vi "SelectMouseRoi.vi"(6 "Refnum in":T1, 7 "Select mouse":bool, 10 "File Path for Mouse Mask":path=path "C:/PassiveRotationTask/MousePositionMask.bmp", 11 "MouseRoi":T1) -> (3 "MouseRoi Out":T1)   [LabVIEW 2013]
uses:
  <vilib>/vision/Image Controls.llb/IMAQ Image.ctl
  <vilib>/vision/NI_Vision_Development_Module.lvlib
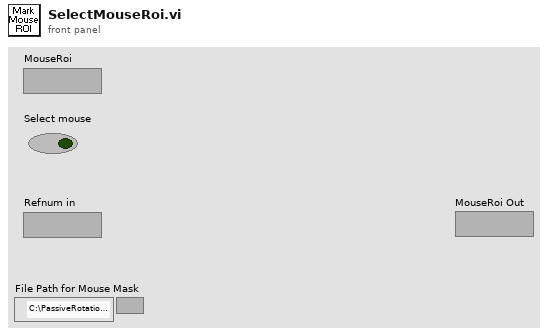
[diagram p1: front panel]
types:
  T1 = typedef "IMAQ Image.ctl" = refnum<image>
  T2 = typedef "ROI Descriptor" = cluster{"Global Rectangle":i32[], "Contours":cluster{"ID":enum32{"External", "Internal"}, "Type":u32, "Coordinates":i32[]}[]}
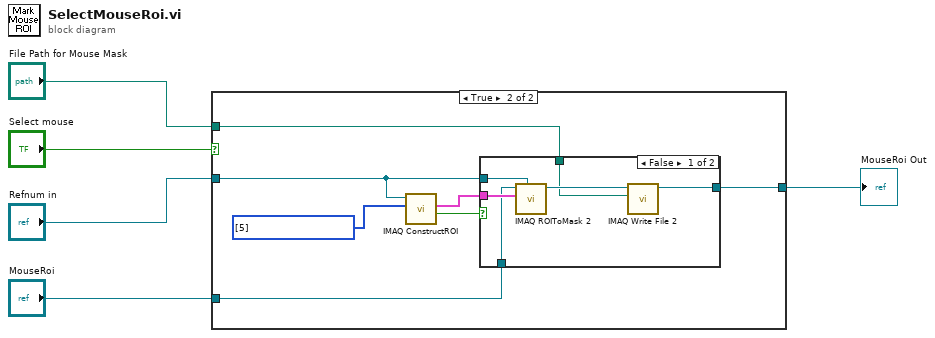
[diagram p0: block diagram]
diagram:
  n1 = case shown="True" "Select mouse" {
    tunnel: "Refnum in" -> [_ w11]
    tunnel: "File Path for Mouse Mask" -> [_ w9]
    tunnel: "MouseRoi" -> [w6 w8]
    tunnel: [w6 w7] -> w1
    frame False {
    }
    frame True {
      w13 = u32[] [5] items=["No Selection", "Point", "Line", "Rectangle", "Oval", "Polygon", "Freehand Region", "Annulus", "Zoom", "Pan", "Broken Line", "Freehand Line", "Rotated Rectangle"] ("Tools")
      n2 = call "IMAQ ConstructROI"("Tools"=w13, "Image"=w11) -> ("Cancel"=w10:bool, "ROI Descriptor Out"=w12:T2)  [unwired: 6 in, 2 out]
      n3 = case shown="False" w10 {
        tunnel: w12 -> [w19 _]
        tunnel: w9 -> [w17 _]
        tunnel: w11 -> [w16 _]
        tunnel: w8 -> [w15 w20]
        tunnel: [w14 w20] -> w7
        frame False {
          n4 = call "IMAQ ROIToMask 2"("Image Model"=w16, "ROI Descriptor"=w19, "Image"=w15) -> ("Image Out"=w18:T1)  [unwired: 6 in, 2 out]
          n5 = call-poly "IMAQ Write File 2"("File Path"=w17, "Image"=w18) -> ("Image Out (duplicate)"=w14:T1)  [unwired: 8 in, 1 out]
        }
        frame True {
        }
      }
    }
  }
  "MouseRoi Out" <- w1
